vi "H5Dcreate.vi"(4 "Dataset Access Property List":T1, 5 "Link Creation Property List":T1, 6 "Dataset Creation Property List":T1, 7 "Name":string, 8 "error in (no error)":errorcluster, 9 "HDF5 Dataspace Ref":T1, 10 "HDF5 Datatype Ref":T1, 11 "HDF5 Location Ref":T1) -> (0 "error out":errorcluster, 2 "HDF5 Dataset Ref":T1, 3 "HDF5 Ref out":T1)   [LabVIEW 2017]
doc: "Creates a new dataset and links it into the file."
uses:
  <vilib>/UPVI/lvhdf5/library.llb/HDF5 Ref.ctl
  <vilib>/UPVI/lvhdf5/hdf5.dll
panel:
  # "LVHDF5 Toolkit\nCopyright (c) 2005-2013 by Jason D. Sommerville\nCopyright (c) 2014 by UPVI, LLC.\n\nThis use and distribution of this file is governed by the terms found in \nLICENSE.txt distributed with this toolkit and installed at\n <user.lib>\\_lvhdf5\\LICENSE.txt"
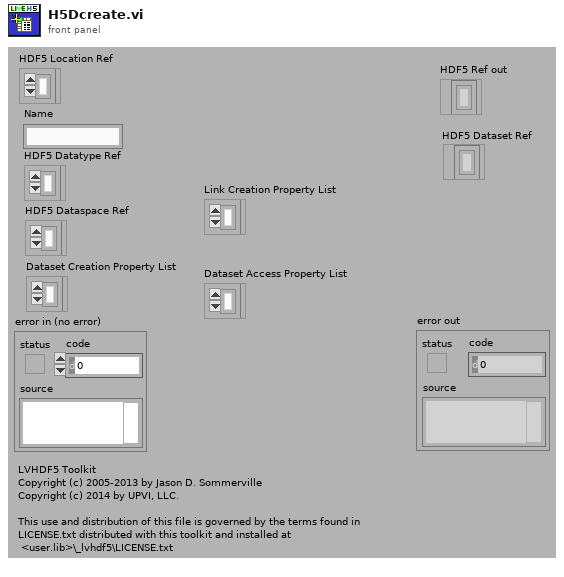
[diagram p1: front panel]
types:
  T1 = typedef "HDF5 Ref.ctl" = refnum<k1>
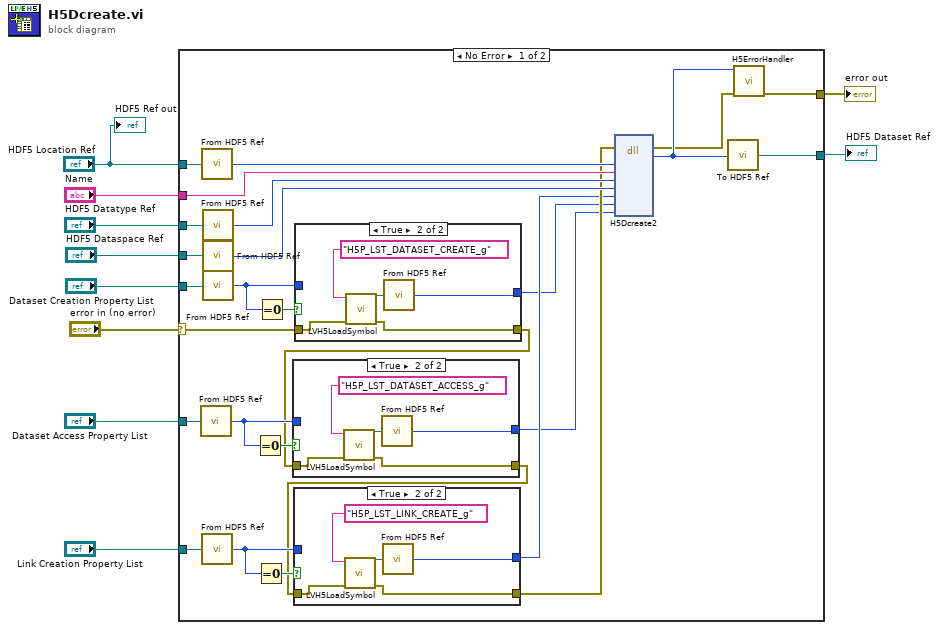
[diagram p0: block diagram]
diagram:
  n1 = case shown="No Error" "error in (no error)" {
    selector: "error in (no error)" -> [w24 w59]
    tunnel: [w37 w59] -> w9
    tunnel: "HDF5 Location Ref" -> [w36 _]
    tunnel: "HDF5 Datatype Ref" -> [w32 _]
    tunnel: "HDF5 Dataspace Ref" -> [w31 _]
    tunnel: "Dataset Creation Property List" -> [w30 _]
    tunnel: "Name" -> [w29 _]
    tunnel: [w27 _] -> w4
    tunnel: "Link Creation Property List" -> [w15 _]
    tunnel: "Dataset Access Property List" -> [w14 _]
    frame No Error {
      n2 = call <vilib>:"From HDF5 Ref.vi"("HDF5 Ref"=w14) -> ("I32"=w22:i32)
      n3 = call <vilib>:"From HDF5 Ref.vi"("HDF5 Ref"=w36) -> ("I32"=w35:i32)
      n4 = call <vilib>:"From HDF5 Ref.vi"("HDF5 Ref"=w15) -> ("I32"=w20:i32)
      n5 = call <vilib>:"From HDF5 Ref.vi"("HDF5 Ref"=w32) -> ("I32"=w34:i32)
      n6 = call <vilib>:"From HDF5 Ref.vi"("HDF5 Ref"=w31) -> ("I32"=w33:i32)
      n7 = call <vilib>:"From HDF5 Ref.vi"("HDF5 Ref"=w30) -> ("I32"=w25:i32)
      n8 = Equal To 0?(x=w22) -> (x = 0?=w23:bool)
      n9 = Equal To 0?(x=w20) -> (x = 0?=w21:bool)
      n10 = Equal To 0?(x=w25) -> (x = 0?=w26:bool)
      n11 = case shown="True" w26 {
        tunnel: w25 -> [w53 _]
        tunnel: w24 -> [w52 w56]
        tunnel: [w53 w58] -> w12
        tunnel: [w52 w55] -> w19
        frame False {
        }
        frame True {
          n12 = call <vilib>:"LVH5LoadSymbol.vi"("error in (no error)"=w56, "Symbol"="H5P_LST_DATASET_CREATE_g") -> ("error out"=w55:errorcluster, "Refnum out"=w54:T1)  [unwired: 8 in]
          n13 = call <vilib>:"From HDF5 Ref.vi"("HDF5 Ref"=w54) -> ("I32"=w58:i32)
        }
      }
      n14 = case shown="True" w23 {
        tunnel: w22 -> [w46 _]
        tunnel: w19 -> [w45 w49]
        tunnel: [w46 w51] -> w11
        tunnel: [w45 w48] -> w18
        frame False {
        }
        frame True {
          n15 = call <vilib>:"LVH5LoadSymbol.vi"("error in (no error)"=w49, "Symbol"="H5P_LST_DATASET_ACCESS_g") -> ("error out"=w48:errorcluster, "Refnum out"=w47:T1)  [unwired: 8 in]
          n16 = call <vilib>:"From HDF5 Ref.vi"("HDF5 Ref"=w47) -> ("I32"=w51:i32)
        }
      }
      n17 = case shown="True" w21 {
        tunnel: w20 -> [w39 _]
        tunnel: w18 -> [w38 w40]
        tunnel: [w39 w44] -> w13
        tunnel: [w38 w42] -> w17
        frame False {
        }
        frame True {
          n18 = call <vilib>:"LVH5LoadSymbol.vi"("error in (no error)"=w40, "Symbol"="H5P_LST_LINK_CREATE_g") -> ("error out"=w42:errorcluster, "Refnum out"=w41:T1)  [unwired: 8 in]
          n19 = call <vilib>:"From HDF5 Ref.vi"("HDF5 Ref"=w41) -> ("I32"=w44:i32)
        }
      }
      n20 = dll-call lib="C:/Program Files/National Instruments/LabVIEW 2017/vi.lib/UPVI/lvhdf5/hdf5.dll" fn="H5Dcreate2" label="H5Dcreate"(error in=w17, "loc_id"=w35, "name"=w29, "type_id"=w34, "space_id"=w33, "lcpl_id"=w13, "dcpl_id"=w12, "dapl_id"=w11) -> (error out=w16:errorcluster, "return type"=w28:i32)  [unwired: 9 in, 1 out]
      n21 = call <vilib>:"To HDF5 Ref.vi"("I32"=w28) -> ("HDF5 Ref"=w27:T1)
      n22 = call <vilib>:"H5ErrorHandler.vi"("error in (no error)"=w16, "herr_t"=w28) -> ("error out"=w37:errorcluster)  [unwired: 3 in, 4 out]
    }
    frame Error {
    }
  }
  "error out" <- w9
  "HDF5 Dataset Ref" <- w4
  "HDF5 Ref out" <- "HDF5 Location Ref"
